vi "Subscribe to Group (SubVI).vi"(8 "error in (no error)":errorcluster, 9 "group":string, 10 "chat id":i32, 11 "first_name":string) -> (0 "error out":errorcluster)   [LabVIEW 2020, in "Notification.lvlib"]
uses:
  Notification.lvlib
  <vilib>/Utility/config.llb/Write Key (I32).vi
  <vilib>/Utility/config.llb/NI_LVConfig.lvlib
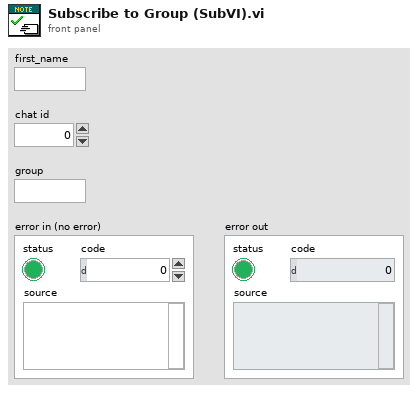
[diagram p1: front panel]
types:
  T1 = typedef "NI_LVConfig.lvlib/Config Data RefNum.ctl" = refnum<k1>
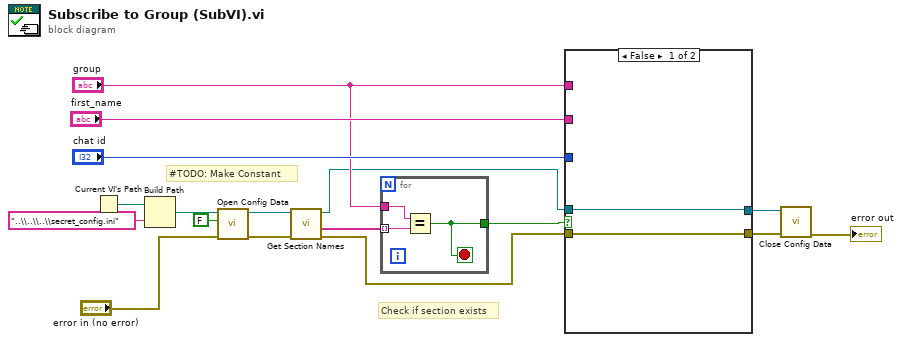
[diagram p0: block diagram]
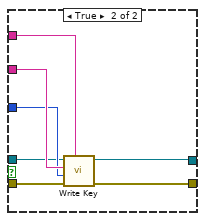
[diagram p2: hidden frame]
diagram:
  # "#TODO: Make Constant"
  # "Check if section exists"
  n1 = Current VI's Path() -> (path=w4:path)
  n2 = Build Path(base path=w4, name or relative path="..\\..\\..\\secret_config.ini") -> (appended path=w2:path)
  n3 = call <vilib>:"Open Config Data.vi"("error in (no error)"="error in (no error)", "create file if necessary (T)"=FALSE, "configuration file path"=w2) -> ("error out"=w14:errorcluster, "refnum"=w13:T1)  [unwired: 6 in, 1 out]
  n4 = call <vilib>:"Get Section Names.vi"("error in (no error)"=w14, "refnum"=w13) -> ("error out"=w9:errorcluster, "section names"=w11:string[], "refnum out"=w6:T1)  [unwired: 7 in]
  n5 = for {
    tunnel: "group" -> [w19]
    tunnel: w11 -> [w20] mode=indexing
    tunnel: [w18] -> w10
    stop <- w18 stop-if-true
    n6 = Equal?(x=w19, y=w20) -> (x = y?=w18:bool)
  }
  n7 = case shown="False" w10 {
    tunnel: "first_name" -> [_ w29]
    tunnel: "chat id" -> [_ w28]
    tunnel: "group" -> [_ w27]
    tunnel: w9 -> [w22 w26]
    tunnel: [w22 w23] -> w8
    tunnel: [w21 w24] -> w7
    tunnel: w6 -> [w21 w25]
    frame False {
    }
    frame True {
      n8 = call-poly <vilib>:"Write Key.vi"("section"=w27, "error in (no error)"=w26, "value"=w28, "key"=w29, "refnum"=w25) -> ("error out"=w23:errorcluster, "refnum out"=w24:T1)  [unwired: 4 in, 1 out]
    }
  }
  n9 = call <vilib>:"Close Config Data.vi"("error in (no error)"=w8, "refnum"=w7) -> ("error out"=→"error out":errorcluster)  [unwired: 8 in, 1 out]
